vi "最终测试报告.vi"(8 "打印?":bool, 11 "报告时间":timestamp) -> ()   [LabVIEW 2010]
uses:
  <vilib>/Utility/NIReport.llb/NI_report.lvclass
  <vilib>/Utility/NIReport.llb/Append Report Text (str wrap).vi
  <vilib>/addons/_office/word.llb/Word Edit Cell ([str]).vi
  <vilib>/addons/_office/NI_ReportGenerationToolkit.lvlib
  <vilib>/Utility/NIReport.llb/Word/NI_Word.lvclass
  全局量/自动测试结果.vi
panel:
  in  "数字量输出":string[][](table)
  in  "数字量输入":string[][](table)
  out "XY图":cluster{"Y":dbl[], "Y":dbl[]}[](graph)
  # "T：打印\nF：保存"
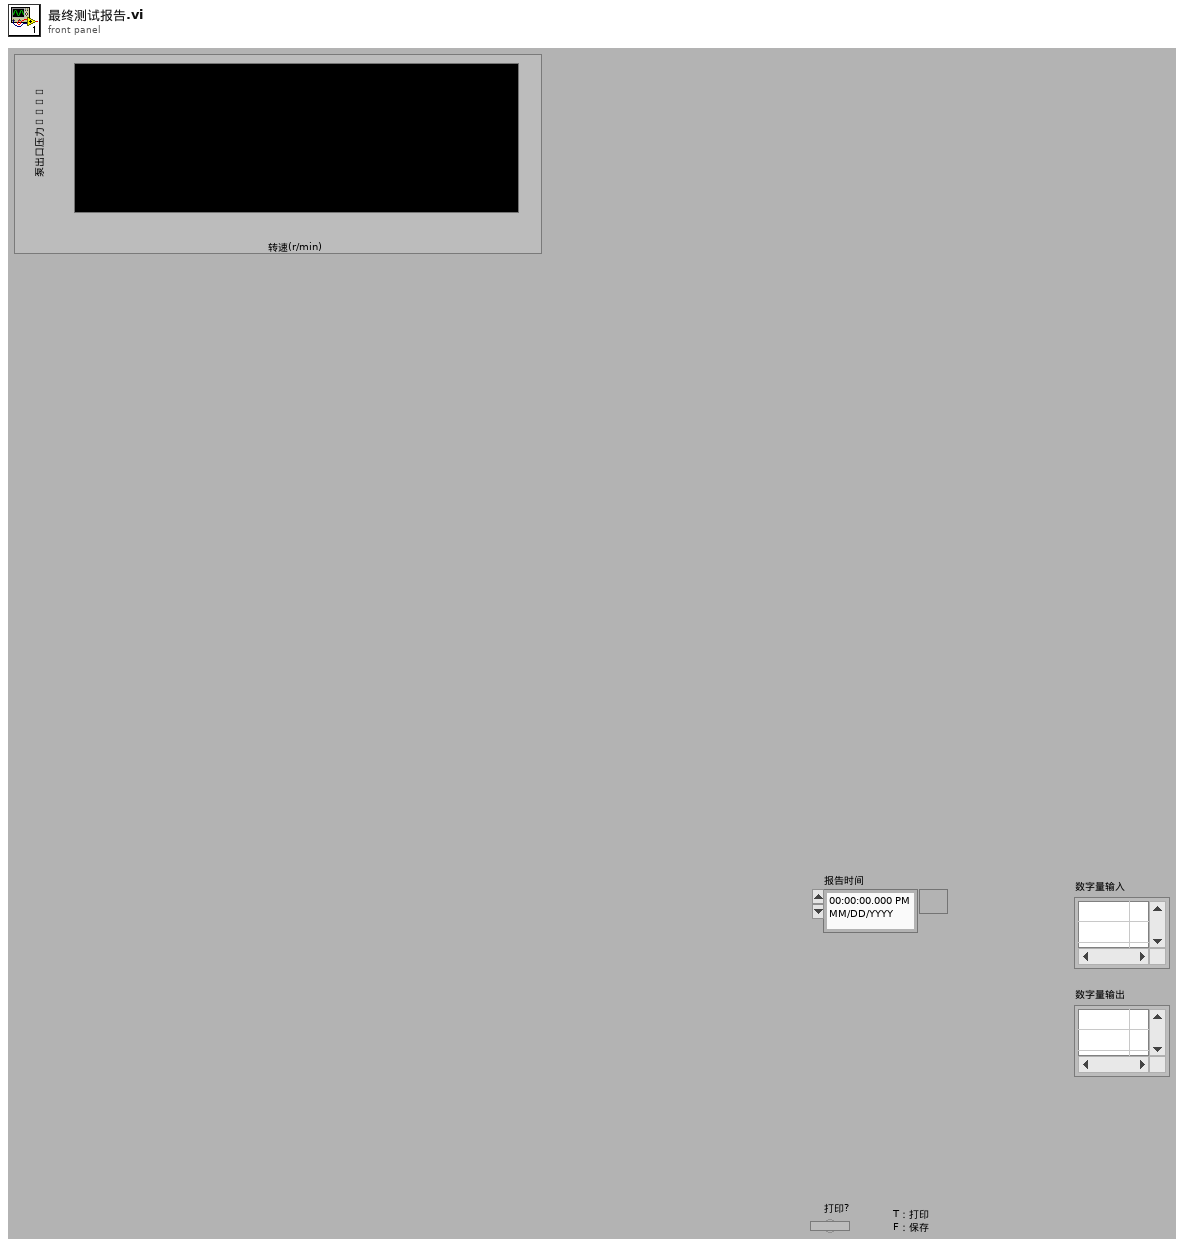
[diagram p1: front panel]
types:
  T1 = cluster{"position (Excel)":cluster{"row":i32, "column":i32}, "name (Excel)":string, "bookmark (Word)":string}
  T2 = enum16{"maximized", "minimized", "normal", "no change"}
  T3 = enum16{"Standard Report", "HTML", "Word", "Excel"}
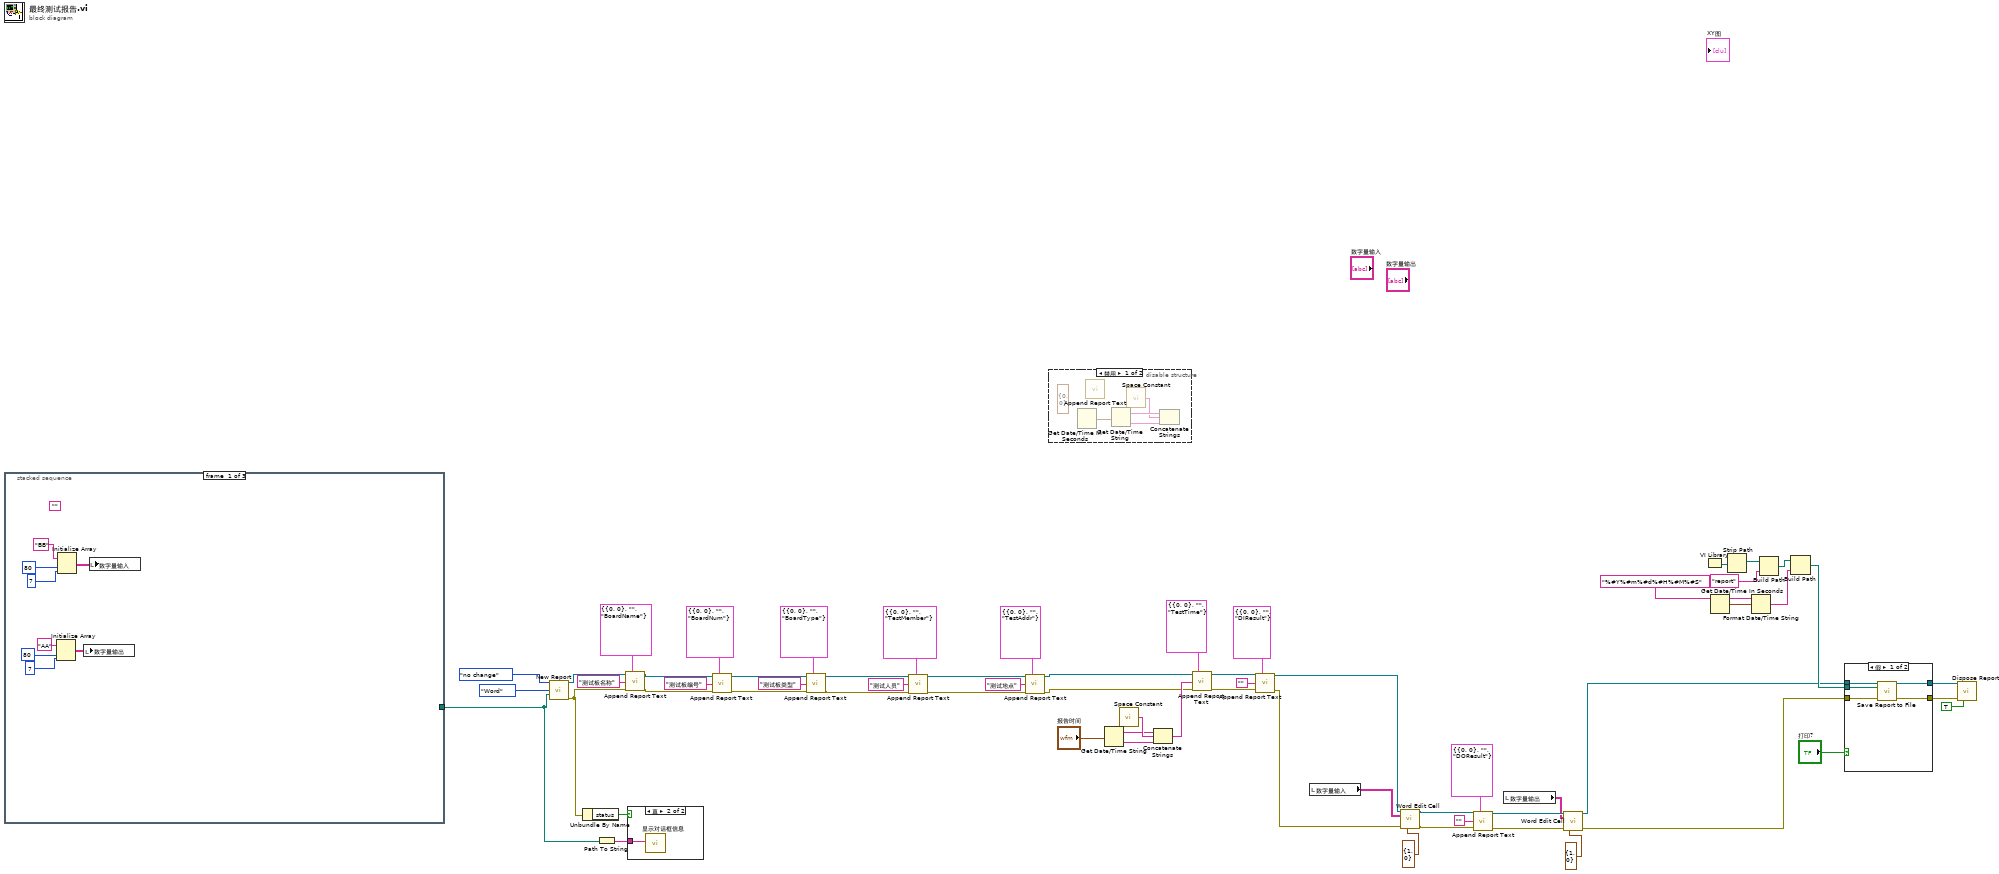
[diagram p0: block diagram]
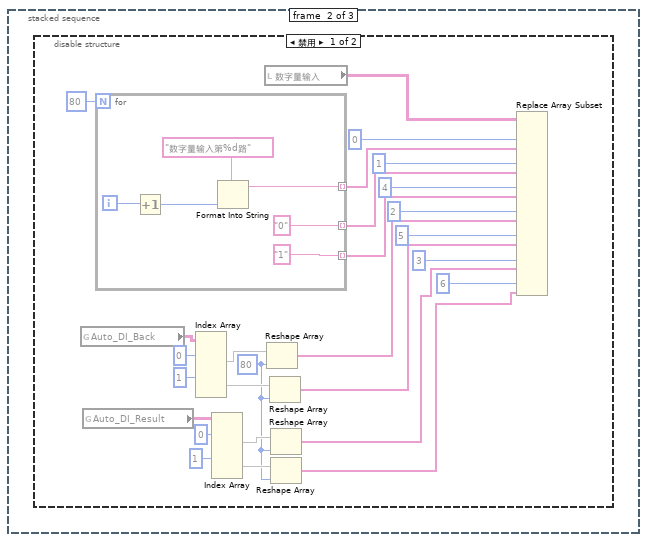
[diagram p2: hidden frame]
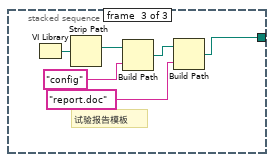
[diagram p4: hidden frame]
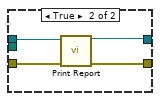
[diagram p5: hidden frame]
diagram:
  n1 = stacked-sequence {
    tunnel: [_ _ w105] -> w15
    frame #0 {
      (unwired) ""
      n2 = Initialize Array("AA", 80 ("维数大小"), 7 ("维数大小")) -> (w65:string[][])
      n3 = Initialize Array("BB", 80 ("维数大小"), 7 ("维数大小")) -> (w69:string[][])
      n4 = local write "数字量输出"(w65) -> ()
      n5 = local write "数字量输入"(w69) -> ()
    }
    frame #1 {
      n6 = disable-structure shown="禁用" {
        frame Disabled {
          w74 = 80 ("维数大小")
          n7 = global read "自动测试结果.vi" "Auto_DI_Back"() -> (w86:string[][][])
          n8 = global read "自动测试结果.vi" "Auto_DI_Result"() -> (w79:string[][][])
          n9 = for {
            N: 80 -> [_]
            tunnel: [w104] -> w95 mode=indexing
            tunnel: ["0"] -> w93 mode=indexing
            tunnel: ["1"] -> w91 mode=indexing
            i -> [w100]
            n10 = Increment(x=w100) -> (x+1=w99:i32)
            n11 = Format Into String(format string="数字量输入第%d路", w99) -> (resulting string=w104:string)  [unwired: 2 in, 1 out]
          }
          n12 = Index Array(array=w86, index (dim 0) #1=0 ("索引 (页)"), index (dim 0) #2=1 ("索引 (页)")) -> (element #1=w83:string[][], element #2=w82:string[][])  [unwired: 4 in]
          n13 = Index Array(array=w79, index (dim 0) #1=0 ("索引 (页)"), index (dim 0) #2=1 ("索引 (页)")) -> (element #1=w76:string[][], element #2=w75:string[][])  [unwired: 4 in]
          n14 = local read "数字量输入"() -> (w97:string[][])
          n15 = Reshape Array(w83, w74) -> (w81:string[])
          n16 = Reshape Array(w82, w74) -> (w80:string[])
          n17 = Reshape Array(w76, w74) -> (w73:string[])
          n18 = Reshape Array(w75, w74) -> (w72:string[])
          n19 = Replace Array Subset(array=w97, new element #1=w95, index (col) #1=0 ("禁用的索引 (列)"), new element #2=w93, index (col) #2=1 ("索引 (列)"), new element #3=w91, index (col) #3=4 ("索引 (列)"), new element #4=w81, index (col) #4=2 ("索引 (列)"), new element #5=w80, index (col) #5=5 ("索引 (列)"), new element #6=w73, index (col) #6=3 ("索引 (列)"), new element #7=w72, index (col) #7=6 ("索引 (列)")) -> ()  [unwired: 7 in, 1 out]
        }
        frame Enabled {
        }
      }
    }
    frame #2 {
      # "试验报告模板"
      n20 = VI Library() -> (path=w110:path)
      n21 = Strip Path(path=w110) -> (stripped path=w107:path)  [unwired: 1 out]
      n22 = Build Path(base path=w107, name or relative path="config") -> (appended path=w109:path)
      n23 = Build Path(base path=w109, name or relative path="report.doc") -> (appended path=w105:path)
    }
  }
  n24 = call <vilib>:"New Report.vi"("window state (normal)"=T2."no change", "report type"=T3."Word", "template (empty)"=w15) -> ("report out"=w48:refnum<class "NI_report.lvclass">, "error out"=w47:errorcluster)  [unwired: 11 in]
  n25 = Unbundle By Name(w47) -> ("status"=w57:bool)
  n26 = Path To String(path=w15) -> (string=w55:string)
  n27 = call-poly <vilib>:"Append Report Text.vi"("report in"=w48, "MS Office parameters"=T1 {"position (Excel)"={"row"=0, "column"=0}, "name (Excel)"="", "bookmark (Word)"="BoardName"}, "text"="测试板名称", "error in (no error)"=w47) -> ("report out"=w36:refnum<class "NI_report.lvclass">, "error out"=w35:errorcluster)  [unwired: 8 in, 2 out]
  n28 = case shown="真" w57 {
    tunnel: w55 -> [_ w111]
    frame False {
    }
    frame True {
      n29 = call "显示对话框信息"("Message"=w111) -> ()  [unwired: 9 in, 2 out]
    }
  }
  n30 = call-poly <vilib>:"Append Report Text.vi"("report in"=w36, "MS Office parameters"=T1 {"position (Excel)"={"row"=0, "column"=0}, "name (Excel)"="", "bookmark (Word)"="BoardNum"}, "text"="测试板编号", "error in (no error)"=w35) -> ("report out"=w32:refnum<class "NI_report.lvclass">, "error out"=w31:errorcluster)  [unwired: 8 in, 2 out]
  n31 = call-poly <vilib>:"Append Report Text.vi"("report in"=w32, "MS Office parameters"=T1 {"position (Excel)"={"row"=0, "column"=0}, "name (Excel)"="", "bookmark (Word)"="BoardType"}, "text"="测试板类型", "error in (no error)"=w31) -> ("report out"=w28:refnum<class "NI_report.lvclass">, "error out"=w27:errorcluster)  [unwired: 8 in, 2 out]
  n32 = call-poly <vilib>:"Append Report Text.vi"("report in"=w28, "MS Office parameters"=T1 {"position (Excel)"={"row"=0, "column"=0}, "name (Excel)"="", "bookmark (Word)"="TestMember"}, "text"="测试人员", "error in (no error)"=w27) -> ("report out"=w24:refnum<class "NI_report.lvclass">, "error out"=w23:errorcluster)  [unwired: 8 in, 2 out]
  n33 = call-poly <vilib>:"Append Report Text.vi"("report in"=w24, "MS Office parameters"=T1 {"position (Excel)"={"row"=0, "column"=0}, "name (Excel)"="", "bookmark (Word)"="TestAddr"}, "text"="测试地点", "error in (no error)"=w23) -> ("report out"=w22:refnum<class "NI_report.lvclass">, "error out"=w21:errorcluster)  [unwired: 8 in, 2 out]
  n34 = disable-structure shown="禁用" {
    frame Disabled {
      (unwired) cluster{"row":i32, "column":i32} {"row"=0, "column"=0} ("position (excel)")
      n35 = Get Date/Time In Seconds() -> (seconds since 1Jan1904=w115:timestamp)
      n36 = call-poly <vilib>:"Append Report Text.vi"() -> ()  [unwired: 12 in, 4 out]
      n37 = Get Date/Time String(seconds (now)=w115) -> (date string=w114:string, time string=w113:string)  [unwired: 2 in]
      n38 = call <vilib>:"Space Constant.vi"() -> ("String"=w112:string)
      n39 = Concatenate Strings(w114, w112, w113) -> ()  [unwired: 1 out]
    }
    frame Enabled {
    }
  }
  n40 = Get Date/Time String(seconds (now)="报告时间") -> (date string=w50:string, time string=w51:string)  [unwired: 2 in]
  n41 = call <vilib>:"Space Constant.vi"() -> ("String"=w52:string)
  n42 = Concatenate Strings(w50, w52, w51) -> (w49:string)
  n43 = call-poly <vilib>:"Append Report Text.vi"("report in"=w22, "MS Office parameters"=T1 {"position (Excel)"={"row"=0, "column"=0}, "name (Excel)"="", "bookmark (Word)"="TestTime"}, "text"=w49, "error in (no error)"=w21) -> ("report out"=w19:refnum<class "NI_report.lvclass">, "error out"=w18:errorcluster)  [unwired: 8 in, 2 out]
  n44 = call-poly <vilib>:"Append Report Text.vi"("report in"=w19, "MS Office parameters"=T1 {"position (Excel)"={"row"=0, "column"=0}, "name (Excel)"="", "bookmark (Word)"="DIResult"}, "text"="", "error in (no error)"=w18) -> ("report out"=w4:refnum<class "NI_report.lvclass">, "error out"=w3:errorcluster)  [unwired: 8 in, 2 out]
  n45 = local read "数字量输入"() -> (w13:string[][])
  n46 = call-poly <vilib>:"Word Edit Cell.vi"("report in"=w4, "value"=w13, "error in (no error)"=w3, "start (0, 0)"=cluster{"row":i32, "column":i32} {"row"=1, "column"=0}) -> ("report out"=w9:refnum<class "NI_report.lvclass">, "error out"=w8:errorcluster)  [unwired: 10 in]
  n47 = call-poly <vilib>:"Append Report Text.vi"("report in"=w9, "MS Office parameters"=T1 {"position (Excel)"={"row"=0, "column"=0}, "name (Excel)"="", "bookmark (Word)"="DOResult"}, "text"="", "error in (no error)"=w8) -> ("report out"=w7:refnum<class "NI_report.lvclass">, "error out"=w6:errorcluster)  [unwired: 8 in, 2 out]
  n48 = local read "数字量输出"() -> (w5:string[][])
  n49 = call-poly <vilib>:"Word Edit Cell.vi"("report in"=w7, "value"=w5, "error in (no error)"=w6, "start (0, 0)"=cluster{"row":i32, "column":i32} {"row"=1, "column"=0}) -> ("report out"=w2:refnum<class "NI_report.lvclass">, "error out"=w1:errorcluster)  [unwired: 10 in]
  n50 = VI Library() -> (path=w58:path)
  n51 = Get Date/Time In Seconds() -> (seconds since 1Jan1904=w46:timestamp)
  n52 = Strip Path(path=w58) -> (stripped path=w61:path)  [unwired: 1 out]
  n53 = Format Date/Time String(time format string (%c)="%#Y%#m%#d%#H%#M%#S" ("时间格式字符串(%c)"), seconds (now)=w46) -> (date/time string=w20:string)  [unwired: 1 in]
  n54 = Build Path(base path=w61, name or relative path="report") -> (appended path=w59:path)
  n55 = Build Path(base path=w59, name or relative path=w20) -> (appended path=w41:path)
  n56 = case shown="假" "打印?" {
    tunnel: w2 -> [w120 w124]
    tunnel: w1 -> [w119 w123]
    tunnel: [w118 w122] -> w44
    tunnel: [w117 w121] -> w43
    tunnel: w41 -> [w116 _]
    frame False {
      n57 = call-dynamic "Save Report to File.vi"("report in"=w120, "report file path"=w116, "error in (no error)"=w119) -> ("report out"=w118:refnum<class "NI_report.lvclass">, "error out"=w117:errorcluster)  [unwired: 11 in]
    }
    frame True {
      n58 = call-dynamic "Print Report.vi"("report in"=w124, "error in (no error)"=w123) -> ("report out"=w122:refnum<class "NI_report.lvclass">, "error out"=w121:errorcluster)  [unwired: 12 in]
    }
  }
  n59 = call-dynamic "Dispose Report.vi"("report in"=w44, "error in (no error)"=w43, "close report? (T)"=TRUE) -> ()  [unwired: 12 in, 1 out]
